vi "Write Tree Control Ref.vi"(8 "error in (no error)":errorcluster, 10 "Tag Tree Reference":refnum<vi>, 11 "Tag Tree In":refnum<class "Tag Tree.lvclass">) -> (0 "error out":errorcluster, 3 "Tag Tree Out":refnum<class "Tag Tree.lvclass">)   [LabVIEW 2020, in "Tree Helpers.lvlib" / "Tag Tree.lvclass"]
uses:
  Tag Tree.lvclass
  Tag Tree.lvclass/Tag Tree.ctl
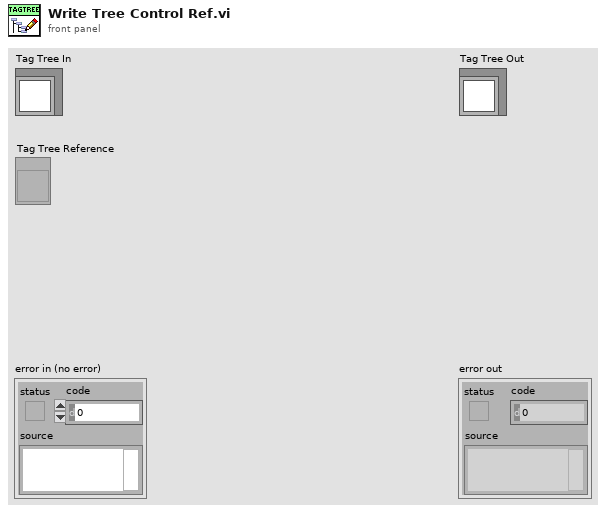
[diagram p1: front panel]
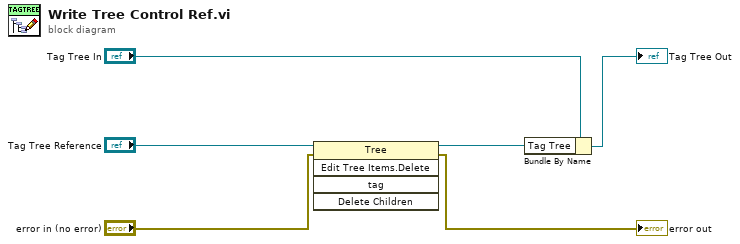
[diagram p0: block diagram]
diagram:
  n1 = invoke class="Tree" method="Edit Tree Items.Delete"(reference="Tag Tree Reference", error in="error in (no error)") -> (reference out=w3:refnum<vi>, error out=→"error out":errorcluster)  [unwired: 3 in, 3 out]
  n2 = Bundle By Name(cluster="Tag Tree In", "Tag Tree"=w3) -> (→"Tag Tree Out":refnum<class "Tag Tree.lvclass">)
